vi "STM Write Meta Data (Serial Ref).vi"(6 "Options":T1={"Ignore Timeout Error"=TRUE, "timeout ms (1000)"=1000}, 7 "Meta data":T2[](array[typedef]), 8 "error in":errorcluster, 11 "VISA resource name":refnum<visa-resource-name>) -> (0 "error out":errorcluster, 3 "Connection Info Out":T3)   [LabVIEW 2014, in "QwaveSys Raspberry Pi Library.lvlib"]
doc: "Use this VI to transmit the meta data cluster to a remote computer. Sending the meta data to another computer helps maintainability since the data resides only on one side and it is shared to other computers at run time."
uses:
  QwaveSys Raspberry Pi Library.lvlib
  stm_Serial Connection Info.ctl
  _SubVIs/stm_MetaDataElement.ctl
  stm_Serial Write Options.ctl
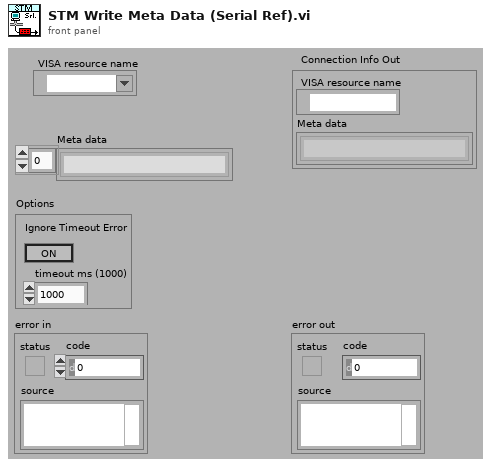
[diagram p1: front panel]
types:
  T1 = typedef "QwaveSys Raspberry Pi Library.lvlib/stm_Serial Write Options.ctl" = cluster{"Ignore Timeout Error":bool, "timeout ms (1000)":u32}
  T2 = typedef "QwaveSys Raspberry Pi Library.lvlib/stm_MetaDataElement.ctl" = string
  T3 = typedef "QwaveSys Raspberry Pi Library.lvlib/stm_Serial Connection Info.ctl" = cluster{"VISA resource name":refnum<visa-resource-name>, "Meta data":T2[]}
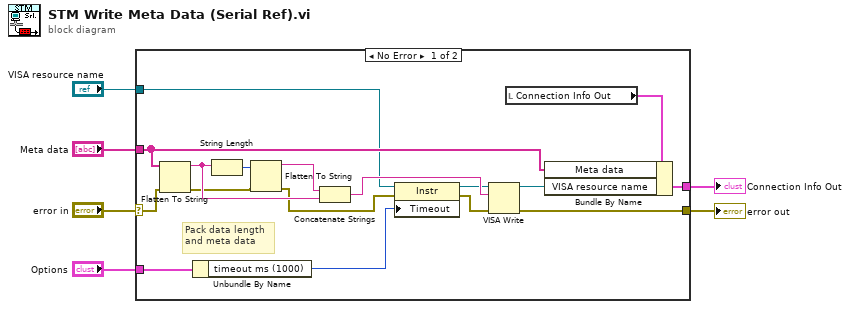
[diagram p0: block diagram]
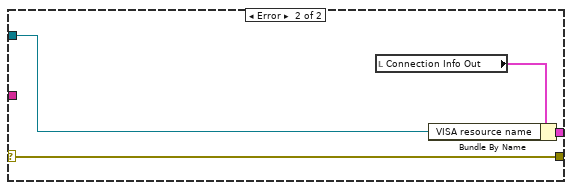
[diagram p2: hidden frame]
diagram:
  n1 = case shown="No Error" "error in" {
    selector: "error in" -> [w14 w27]
    tunnel: [w16 w25] -> w6
    tunnel: "VISA resource name" -> [w11 w24]
    tunnel: "Meta data" -> [w15 _]
    tunnel: [w23 w27] -> w4
    tunnel: "Options" -> [w18 _]
    frame No Error {
      # "Pack data length\nand meta data"
      n2 = Flatten To String(anything=w15, error in (no error)=w14) -> (data string=w19:string, error out=w13:errorcluster)  [unwired: 3 out]
      n3 = Unbundle By Name(w18) -> ("timeout ms (1000)"=w9:u32)
      n4 = String Length(string=w19) -> (length=w22:i32)
      n5 = Flatten To String(anything=w22, error in (no error)=w13) -> (data string=w21:string, error out=w8:errorcluster)  [unwired: 3 out]
      n6 = Concatenate Strings(w21, w19) -> (w20:string)
      n7 = property class="Instr"(reference=w11, error in=w8, "Timeout"=w9) -> (reference out=w10:refnum<visa-resource-name>, error out=w7:errorcluster)
      n8 = VISA Write(VISA resource name=w10, write buffer=w20, error in (no error)=w7) -> (VISA resource name out=w17:refnum<visa-resource-name>, error out=w23:errorcluster)  [unwired: 1 out]
      n9 = local read "Connection Info Out"() -> (w12:T3)
      n10 = Bundle By Name(cluster=w12, "Meta data"=w15, "VISA resource name"=w17) -> (w16:T3)
    }
    frame Error {
      n11 = local read "Connection Info Out"() -> (w26:T3)
      n12 = Bundle By Name(cluster=w26, "VISA resource name"=w24) -> (w25:T3)
    }
  }
  "Connection Info Out" <- w6
  "error out" <- w4
